vi "xy振镜移动.vi"(4 "比例因子(V/°)":dbl=0.5, 5 "速度(°/s)":dbl=0.1, 6 "AO通道：X前Y后":tag="Dev1/ao0:1", 7 "Y初始角(°)":dbl, 8 "X初始角(°)":dbl, 9 "Y终止角(°)":dbl=1.0, 10 "X终止角(°)":dbl=1.0) -> (2 "Y终止角(°) 2":dbl=1.0, 3 "X终止角(°) 2":dbl=1.0)   [LabVIEW 2015]
doc: "速度为0时执行G0指令，可无需连接XY初始角"
uses:
  <vilib>/Platform/TimedLoop/XDataNode/timing_clust.ctl
  <vilib>/Platform/TimedLoop/XDataNode/nitl_modes.ctl
  <vilib>/Platform/TimedLoop/XDataNode/wakeup.ctl
  <vilib>/DAQmx/write.llb/DAQmx Write (Analog 1D DBL NChan 1Samp).vi
  <vilib>/DAQmx/write.llb/DAQmx Write (Analog DBL 1Chan 1Samp).vi
  <vilib>/DAQmx/create/channels.llb/DAQmx Create Channel (AO-Voltage-Basic).vi
  <vilib>/DAQmx/miscellaneous.llb/DAQmx Fill In Error Info.vi
  <vilib>/Platform/TimedLoop/XDataNode/XDataNode.xnode
  <vilib>/Platform/TimedLoop/XDataNode/XDNodeRunTimeDep.lvlib
panel:
  out "移动次数-x":i32
  out "步进-x(°)":dbl
  out "步进-xy-y(°)":dbl
  out "步进-xy-x(°)":dbl
  out "移动次数-xy":i32
  in  "AO通道：单通道":tag="Dev1/ao0:1"
  in  "dt(ms)":i32=100
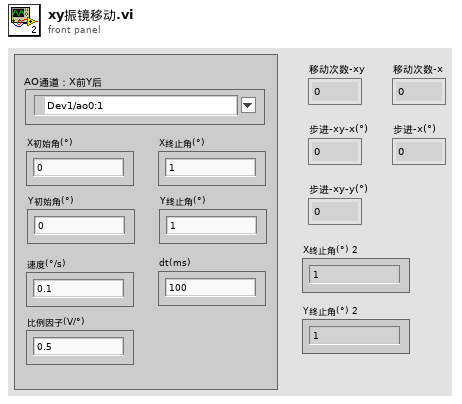
[diagram p1: front panel]
types:
  T1 = typedef "XDNodeRunTimeDep.lvlib/timing_clust.ctl" = cluster{"Expected End [f-1]":u64, "Actual End [f-1]":u64, "Finished Late? [f-1]":bool, "Expected End [i-1]":u64, "Actual End [i-1]":u64, "Finished Late? [i-1]":bool, "Expected Start [i]":u64, "Actual Start [i]":u64, "Expected Start [f]":u64, "Actual Start [f]":u64, "Source Name":string, "Structure Name":string, "Period":i64, "Deadline":i64, "Offset":i64, "Start":i64, "Priority":i32, "Timeout":i32, "Mode":T2, "Wakeup Reason":T3, "Error":errorcluster, "Source Type":string, "Secondary Source Type":string, "Global End Time":u64, "Global Start Time":u64, "Frame Duration":u64, "Iteration Duration":u64, "Assigned CPU":i32, "I/O Scan Engine Mode":u32}
  T2 = typedef "XDNodeRunTimeDep.lvlib/nitl_modes.ctl" = enum32{"No Change", "Process missed periods, maintain original phase", "Discard missed periods, maintain original phase", "Process missed periods, ignore original phase", "Discard missed periods, ignore original phase"}
  T3 = typedef "XDNodeRunTimeDep.lvlib/wakeup.ctl" = enum32{"Normal", "Aborted", "Asynchronous wakeup", "Timing source error", "Timed loop error", "Timeout"}
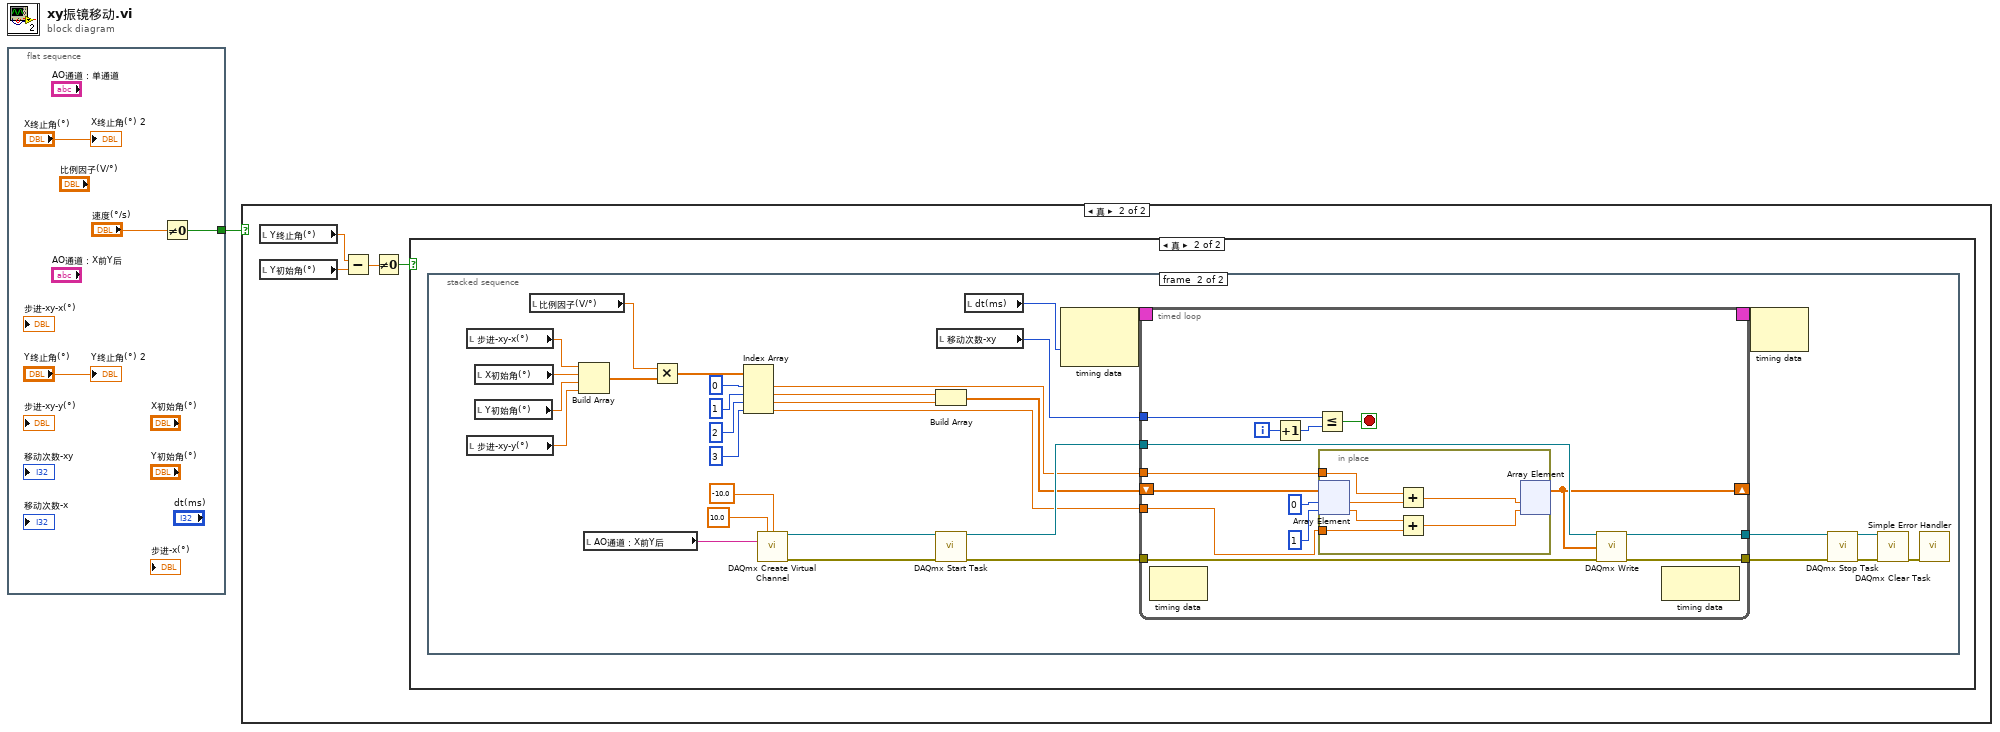
[diagram p0: block diagram]
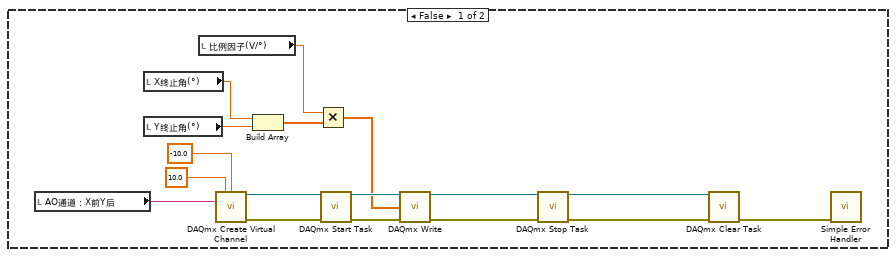
[diagram p2: hidden frame]
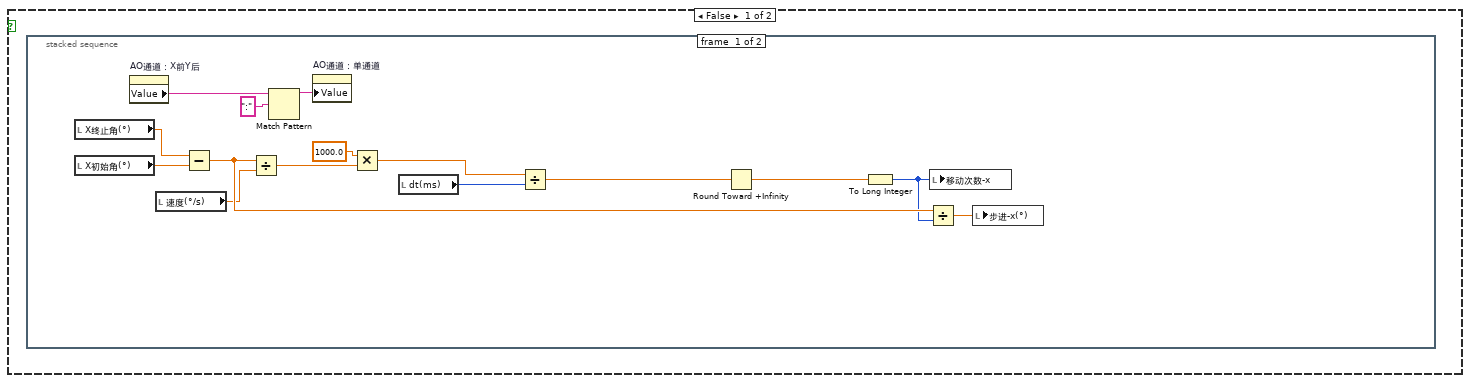
[diagram p3: hidden frame]
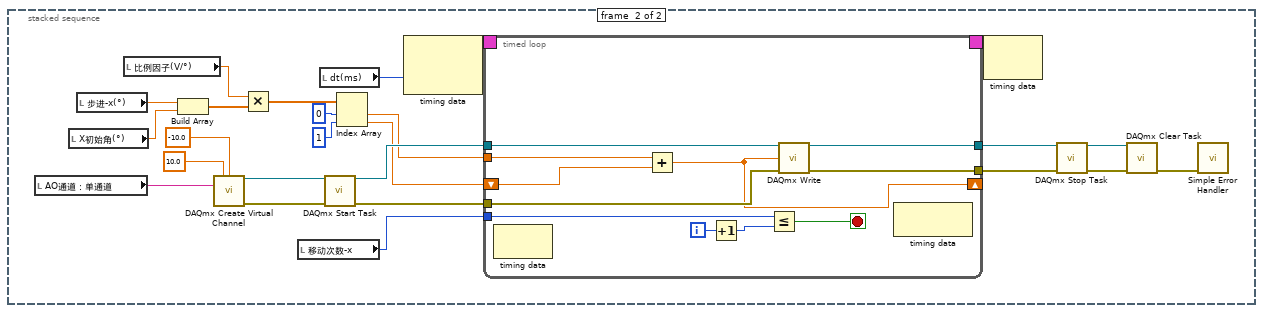
[diagram p4: hidden frame]
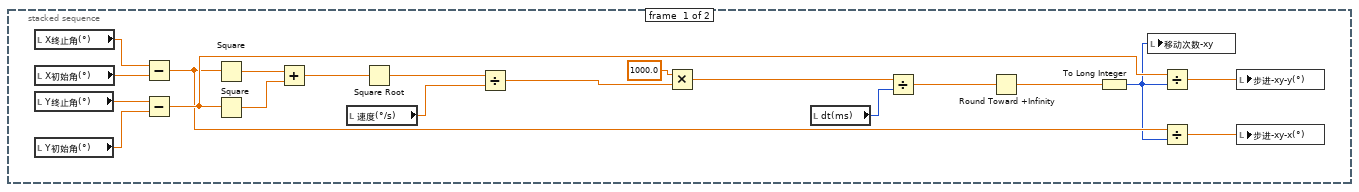
[diagram p5: hidden frame]
diagram:
  n1 = flat-sequence {
    tunnel: [w5] -> w1
    frame #0 {
      n2 = Not Equal To 0?(x="速度(°/s)") -> (x != 0?=w5:bool)
      "X终止角(°) 2" <- "X终止角(°)"
      "Y终止角(°) 2" <- "Y终止角(°)"
    }
  }
  n3 = case shown="真" w1 {
    frame False {
      n4 = local read "AO通道：X前Y后"() -> (w6:tag)
      n5 = local read "X终止角(°)"() -> (w8:dbl)
      n6 = local read "Y终止角(°)"() -> (w9:dbl)
      n7 = local read "比例因子(V/°)"() -> (w7:dbl)
      n8 = call-poly <vilib>:"DAQmx Create Virtual Channel.vi"("maximum value"=10.0, "minimum value"=-10.0, "physical channels"=w6) -> ("task out"=w21:refnum<k21>, "error out"=w20:errorcluster)  [unwired: 11 in]
      n9 = Build Array(w8, w9) -> (w14:dbl[])
      n10 = Multiply(x=w7, y=w14) -> (x*y=w13:dbl[])
      n11 = call <vilib>:"DAQmx Start Task.vi"("task/channels in"=w21, "error in"=w20) -> ("task out"=w15:refnum<k21>, "error out"=w10:errorcluster)  [unwired: 12 in]
      n12 = call-poly <vilib>:"DAQmx Write.vi"("task/channels in"=w15, "data"=w13, "error in"=w10) -> ("task out"=w12:refnum<k21>, "error out"=w11:errorcluster)  [unwired: 10 in, 1 out]
      n13 = call <vilib>:"DAQmx Stop Task.vi"("task/channels in"=w12, "error in"=w11) -> ("task out"=w19:refnum<k21>, "error out"=w18:errorcluster)  [unwired: 12 in]
      n14 = call <vilib>:"DAQmx Clear Task.vi"("task in"=w19, "error in"=w18) -> ("error out"=w22:errorcluster)  [unwired: 13 in]
      n15 = call <vilib>:"Simple Error Handler.vi"("error in (no error)"=w22) -> ()  [unwired: 4 in, 5 out]
    }
    frame True {
      n16 = local read "Y终止角(°)"() -> (w24:dbl)
      n17 = local read "Y初始角(°)"() -> (w23:dbl)
      n18 = Subtract(x=w24, y=w23) -> (x-y=w26:dbl)
      n19 = Not Equal To 0?(x=w26) -> (x != 0?=w25:bool)
      n20 = case shown="真" w25 {
        frame False {
          n21 = stacked-sequence {
            frame #0 {
              n22 = local read "X终止角(°)"() -> (w30:dbl)
              n23 = local read "X初始角(°)"() -> (w35:dbl)
              n24 = property on="AO通道：X前Y后" class="DAQmxName"() -> ("Value"=w31:string)  [unwired: 2 in, 2 out]
              n25 = local read "速度(°/s)"() -> (w29:dbl)
              n26 = Subtract(x=w30, y=w35) -> (x-y=w36:dbl)
              n27 = Divide(x=w36, y=w29) -> (x/y=w39:dbl)
              n28 = Match Pattern(string=w31, regular expression=":" ("正则表达式")) -> (before substring=w33:string)  [unwired: 1 in, 3 out]
              n29 = property on="AO通道：单通道" class="DAQmxName"("Value"=w33) -> ()  [unwired: 2 in, 2 out]
              n30 = Multiply(x=1000.0, y=w39) -> (x*y=w37:dbl)
              n31 = local read "dt(ms)"() -> (w34:i32)
              n32 = Divide(x=w37, y=w34) -> (x/y=w41:dbl)
              n33 = Round Toward +Infinity(x=w41) -> (ceil(x): smallest int >= x=w40:dbl)
              n34 = To Long Integer(number=w40) -> (32bit integer=w27:i32)
              n35 = Divide(x=w36, y=w27) -> (x/y=w28:dbl)
              n36 = local write "移动次数-x"(w27) -> ()
              n37 = local write "步进-x(°)"(w28) -> ()
            }
            frame #1 {
              n38 = local read "AO通道：单通道"() -> (w45:tag)
              n39 = local read "X初始角(°)"() -> (w48:dbl)
              n40 = local read "步进-x(°)"() -> (w42:dbl)
              n41 = local read "比例因子(V/°)"() -> (w44:dbl)
              n42 = Build Array(w42, w48) -> (w52:dbl[])
              n43 = call-poly <vilib>:"DAQmx Create Virtual Channel.vi"("maximum value"=10.0, "minimum value"=-10.0, "physical channels"=w45) -> ("task out"=w63:refnum<k21>, "error out"=w62:errorcluster)  [unwired: 11 in]
              n44 = Multiply(x=w44, y=w52) -> (x*y=w51:dbl[])
              n45 = local read "移动次数-x"() -> (w43:i32)
              n46 = local read "dt(ms)"() -> (w55:i32)
              n47 = call <vilib>:"DAQmx Start Task.vi"("task/channels in"=w63, "error in"=w62) -> ("task out"=w61:refnum<k21>, "error out"=w60:errorcluster)  [unwired: 12 in]
              n48 = Index Array(array=w51, index #1=0 ("索引"), index #2=1 ("索引")) -> (element #1=w47:dbl, element #2=w46:dbl)
              n49 = node-c288(w55) -> (w66:T1)  [unwired: 1 in]
              n50 = timed-loop {
                tunnel: w61 -> [w77]
                tunnel: w60 -> [w75]
                tunnel: [w74] -> w58
                tunnel: [w76] -> w59
                timing: w66 -> [_]
                timing-out: [_] -> w65
                tunnel: w43 -> [w71]
                shift-right: [w67] -> _
                shift-left: w46 -> [w68]
                tunnel: w47 -> [w70]
                i -> [w73]
                stop <- w69 stop-if-true
                n51 = node-c288() -> ()  [unwired: 1 in, 1 out]
                n52 = Add(x=w70, y=w68) -> (x+y=w67:dbl)
                n53 = Increment(x=w73) -> (x+1=w72:i32)
                n54 = Less Or Equal?(x=w71, y=w72) -> (x <= y?=w69:bool)
                n55 = call-poly <vilib>:"DAQmx Write.vi"("task/channels in"=w77, "data"=w67, "error in"=w75) -> ("task out"=w76:refnum<k21>, "error out"=w74:errorcluster)  [unwired: 10 in, 1 out]
                n56 = node-c288() -> ()  [unwired: 1 in, 1 out]
              }
              n57 = node-c288(w65) -> ()  [unwired: 1 out]
              n58 = call <vilib>:"DAQmx Stop Task.vi"("task/channels in"=w59, "error in"=w58) -> ("task out"=w57:refnum<k21>, "error out"=w56:errorcluster)  [unwired: 12 in]
              n59 = call <vilib>:"DAQmx Clear Task.vi"("task in"=w57, "error in"=w56) -> ("error out"=w64:errorcluster)  [unwired: 13 in]
              n60 = call <vilib>:"Simple Error Handler.vi"("error in (no error)"=w64) -> ()  [unwired: 4 in, 5 out]
            }
          }
        }
        frame True {
          n61 = stacked-sequence {
            frame #0 {
              n62 = local read "X终止角(°)"() -> (w91:dbl)
              n63 = local read "X初始角(°)"() -> (w88:dbl)
              n64 = local read "Y终止角(°)"() -> (w90:dbl)
              n65 = local read "Y初始角(°)"() -> (w92:dbl)
              n66 = Subtract(x=w91, y=w88) -> (x-y=w93:dbl)
              n67 = Subtract(x=w90, y=w92) -> (x-y=w94:dbl)
              n68 = Square(x=w93) -> (x^2=w100:dbl)
              n69 = Square(x=w94) -> (x^2=w101:dbl)
              n70 = Add(x=w100, y=w101) -> (x+y=w102:dbl)
              n71 = local read "速度(°/s)"() -> (w89:dbl)
              n72 = Square Root(x=w102) -> (sqrt(x)=w103:dbl)
              n73 = Divide(x=w103, y=w89) -> (x/y=w97:dbl)
              n74 = Multiply(x=1000.0, y=w97) -> (x*y=w95:dbl)
              n75 = local read "dt(ms)"() -> (w85:i32)
              n76 = Divide(x=w95, y=w85) -> (x/y=w99:dbl)
              n77 = Round Toward +Infinity(x=w99) -> (ceil(x): smallest int >= x=w98:dbl)
              n78 = To Long Integer(number=w98) -> (32bit integer=w84:i32)
              n79 = local write "移动次数-xy"(w84) -> ()
              n80 = Divide(x=w94, y=w84) -> (x/y=w86:dbl)
              n81 = Divide(x=w93, y=w84) -> (x/y=w87:dbl)
              n82 = local write "步进-xy-y(°)"(w86) -> ()
              n83 = local write "步进-xy-x(°)"(w87) -> ()
            }
            frame #1 {
              n84 = local read "步进-xy-x(°)"() -> (w104:dbl)
              n85 = local read "步进-xy-y(°)"() -> (w110:dbl)
              n86 = local read "X初始角(°)"() -> (w105:dbl)
              n87 = local read "Y初始角(°)"() -> (w106:dbl)
              n88 = local read "比例因子(V/°)"() -> (w112:dbl)
              n89 = Build Array(w104, w105, w106, w110) -> (w121:dbl[])
              n90 = local read "AO通道：X前Y后"() -> (w113:tag)
              n91 = Multiply(x=w112, y=w121) -> (x*y=w120:dbl[])
              n92 = Index Array(array=w120, index #1=0 ("索引"), index #2=1 ("索引"), index #3=2 ("索引"), index #4=3 ("索引")) -> (element #1=w107:dbl, element #2=w108:dbl, element #3=w109:dbl, element #4=w114:dbl)
              n93 = call-poly <vilib>:"DAQmx Create Virtual Channel.vi"("maximum value"=10.0, "minimum value"=-10.0, "physical channels"=w113) -> ("task out"=w132:refnum<k21>, "error out"=w131:errorcluster)  [unwired: 11 in]
              n94 = Build Array(w108, w109) -> (w117:dbl[])
              n95 = call <vilib>:"DAQmx Start Task.vi"("task/channels in"=w132, "error in"=w131) -> ("task out"=w130:refnum<k21>, "error out"=w129:errorcluster)  [unwired: 12 in]
              n96 = local read "移动次数-xy"() -> (w111:i32)
              n97 = local read "dt(ms)"() -> (w124:i32)
              n98 = node-c288(w124) -> (w135:T1)  [unwired: 1 in]
              n99 = timed-loop {
                tunnel: w130 -> [w146]
                tunnel: w129 -> [w144]
                tunnel: [w143] -> w127
                tunnel: [w145] -> w128
                timing: w135 -> [_]
                timing-out: [_] -> w134
                shift-right: [w138] -> _
                shift-left: w117 -> [w147]
                tunnel: w107 -> [w140]
                tunnel: w114 -> [w139]
                tunnel: w111 -> [w136]
                i -> [w142]
                stop <- w137 stop-if-true
                n100 = node-c288() -> ()  [unwired: 1 in, 1 out]
                n101 = Increment(x=w142) -> (x+1=w141:i32)
                n102 = Less Or Equal?(x=w136, y=w141) -> (x <= y?=w137:bool)
                n103 = in-place {
                  in-place-border: w140 -> [w152]
                  in-place-border: w139 -> [w154]
                  n104 = in-place-array #1(w147, 0, 1) -> (w155:dbl, w153:dbl)
                  n105 = Add(x=w152, y=w155) -> (x+y=w151:dbl)
                  n106 = Add(x=w153, y=w154) -> (x+y=w150:dbl)
                  n107 = in-place-array #1(w151, w150) -> (w138:dbl[])  [unwired: 2 out]
                }
                n108 = call-poly <vilib>:"DAQmx Write.vi"("task/channels in"=w146, "data"=w138, "error in"=w144) -> ("task out"=w145:refnum<k21>, "error out"=w143:errorcluster)  [unwired: 10 in, 1 out]
                n109 = node-c288() -> ()  [unwired: 1 in, 1 out]
              }
              n110 = node-c288(w134) -> ()  [unwired: 1 out]
              n111 = call <vilib>:"DAQmx Stop Task.vi"("task/channels in"=w128, "error in"=w127) -> ("task out"=w126:refnum<k21>, "error out"=w125:errorcluster)  [unwired: 12 in]
              n112 = call <vilib>:"DAQmx Clear Task.vi"("task in"=w126, "error in"=w125) -> ("error out"=w133:errorcluster)  [unwired: 13 in]
              n113 = call <vilib>:"Simple Error Handler.vi"("error in (no error)"=w133) -> ()  [unwired: 4 in, 5 out]
            }
          }
        }
      }
    }
  }
